vi "836_CameraGet Image.vi"(6 "Video Mode":i32, 8 "error in (no error)":errorcluster, 10 "Image":T1, 11 "CameraDevRef":T2={"Camera Address"="192.168.0.90", "CameraStatus"={"status"=FALSE, "code"=0, "source"=""}}) -> (0 "error out":errorcluster, 2 "Image Out":T1, 3 "CameraDevRef Out":T2)   [LabVIEW 2015]
doc: "Retrieves a specific image from the image data that the camera you specify acquired. Use the Start VI to start acquiring image data from the camera before you use the Get Image VI to retrieve an image. When you run this VI, this VI retrieves the most current snapshot of the image data from the camera.\n\nThis software is licensed. Open the labview\\readme\\WPI Robotics Library Open Source License.txt file for more information."
uses:
  <vilib>/Rock Robotics/WPI/Camera/WPI_CameraDevRef.ctl
  <vilib>/vision/Image Controls.llb/IMAQ Image.ctl
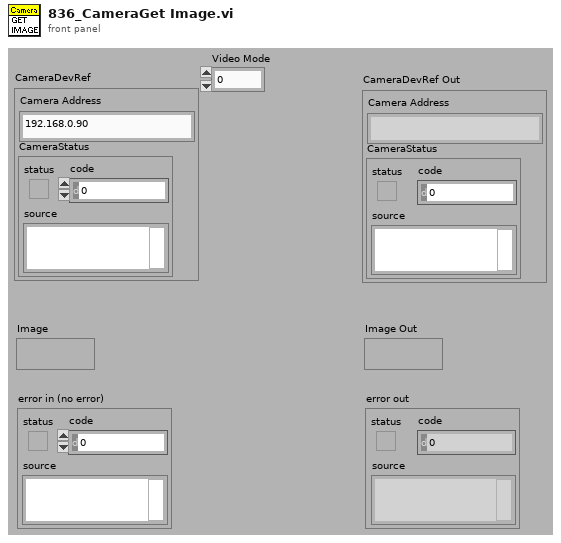
[diagram p1: front panel]
types:
  T1 = typedef "IMAQ Image.ctl" = refnum<image>
  T2 = typedef "WPI_CameraDevRef.ctl" = cluster{"Camera Address":string, "CameraStatus":errorcluster}
  T3 = enum16{"Update Mode", "Get Image", "Get Image Data"}
  T4 = typedef "WPI_CameraFrameRate.ctl" = u32
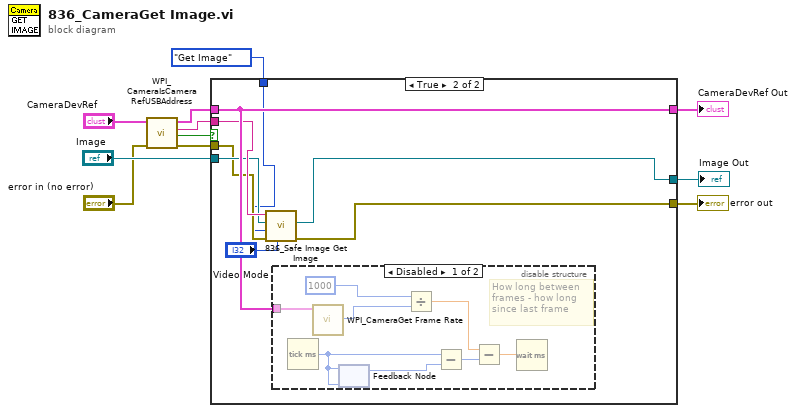
[diagram p0: block diagram]
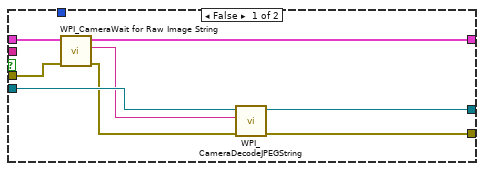
[diagram p2: hidden frame]
diagram:
  n1 = call <vilib>:"WPI_CameraIsCameraRefUSBAddress.vi"("error in (no error)"="error in (no error)", "CameraDevRef"="CameraDevRef") -> ("error out"=w6:errorcluster, "USB?"=w5:bool, "Camera Address Out"=w4:string, "CameraDevRef out"=w2:T2)  [unwired: 6 in]
  n2 = case shown="True" w5 {
    tunnel: "Image" -> [w19 w25]
    tunnel: [w18 w23] -> w10
    tunnel: [w17 w22] -> w9
    tunnel: w2 -> [w15 w27]
    tunnel: [w14 w27] -> w8
    tunnel: w4 -> [_ w26]
    tunnel: w6 -> [w12 w24]
    tunnel: T3."Get Image" ("Operation") -> [_ w21]
    frame False {
      n3 = call <vilib>:"WPI_CameraWait for Raw Image String.vi"("error in (no error)"=w12, "CameraDevRef"=w15) -> ("error out"=w16:errorcluster, "String"=w13:string, "CameraDevRef Out"=w14:T2)  [unwired: 3 in, 4 out]
      n4 = call <vilib>:"WPI_CameraDecodeJPEGString.vi"("error in"=w16, "Compressed Image"=w13, "Image In"=w19) -> ("error out"=w17:errorcluster, "Image Out"=w18:T1)  [unwired: 3 out]
    }
    frame True {
      n5 = call "836_Safe Image Get Image.vi"("Video Mode"="Video Mode", "error in"=w24, "Operation"=w21, "Image In"=w25, "Session In"=w26) -> ("error out"=w22:errorcluster, "Image Out"=w23:T1)  [unwired: 3 in, 2 out]
      n6 = disable-structure shown="Disabled" {
        disable-tunnel: w27 -> [w31 _]
        frame Disabled {
          # "How long between\nframes - how long\nsince last frame"
          n7 = Tick Count (ms)() -> (millisecond timer value=w34:u32)
          n8 = call <vilib>:"WPI_CameraGet Frame Rate.vi"("CameraDevRef"=w31) -> ("Frame Rate (fps)"=w32:T4)  [unwired: 8 in, 2 out]
          n9 = feedback #1(w34) -> (w35:u32)
          n10 = feedback-in #1(w34) -> ()
          n11 = Divide(x=1000, y=w32) -> (x/y=w29:dbl)
          n12 = Subtract(x=w34, y=w35) -> (x-y=w30:u32)
          n13 = Subtract(x=w29, y=w30) -> (x-y=w28:dbl)
          n14 = Wait (ms)(milliseconds to wait=w28) -> ()  [unwired: 1 out]
        }
        frame Enabled {
        }
      }
    }
  }
  "CameraDevRef Out" <- w8
  "Image Out" <- w10
  "error out" <- w9
